vi "Build Msgs.vi"(8 "error in (no error)":errorcluster, 9 "Messages in":map{string, T3}(c390), 10 "Segments in":T1[](array[typedef]), 11 "ProtoParser in":refnum<class "ProtoParser.lvclass">) -> (0 "error out":errorcluster, 1 "Messages":map{string, T3}(c390), 2 "Segments":T1[](array[typedef]), 3 "ProtoParser out":refnum<class "ProtoParser.lvclass">)   [LabVIEW 2020, in "LV-Protoc.lvlib" / "ProtoParser.lvclass"]
uses:
  ProtoParser.lvclass
  Segment Type.ctl
  LV-Protoc.lvlib
  Raw Segment.ctl
  LV-Proto/Proto Type.ctl
  LV-Proto/LV-Proto.lvlib
  LV-Proto/Field.ctl
  LV-Proto/Message.ctl
  LV-Proto/Type.ctl
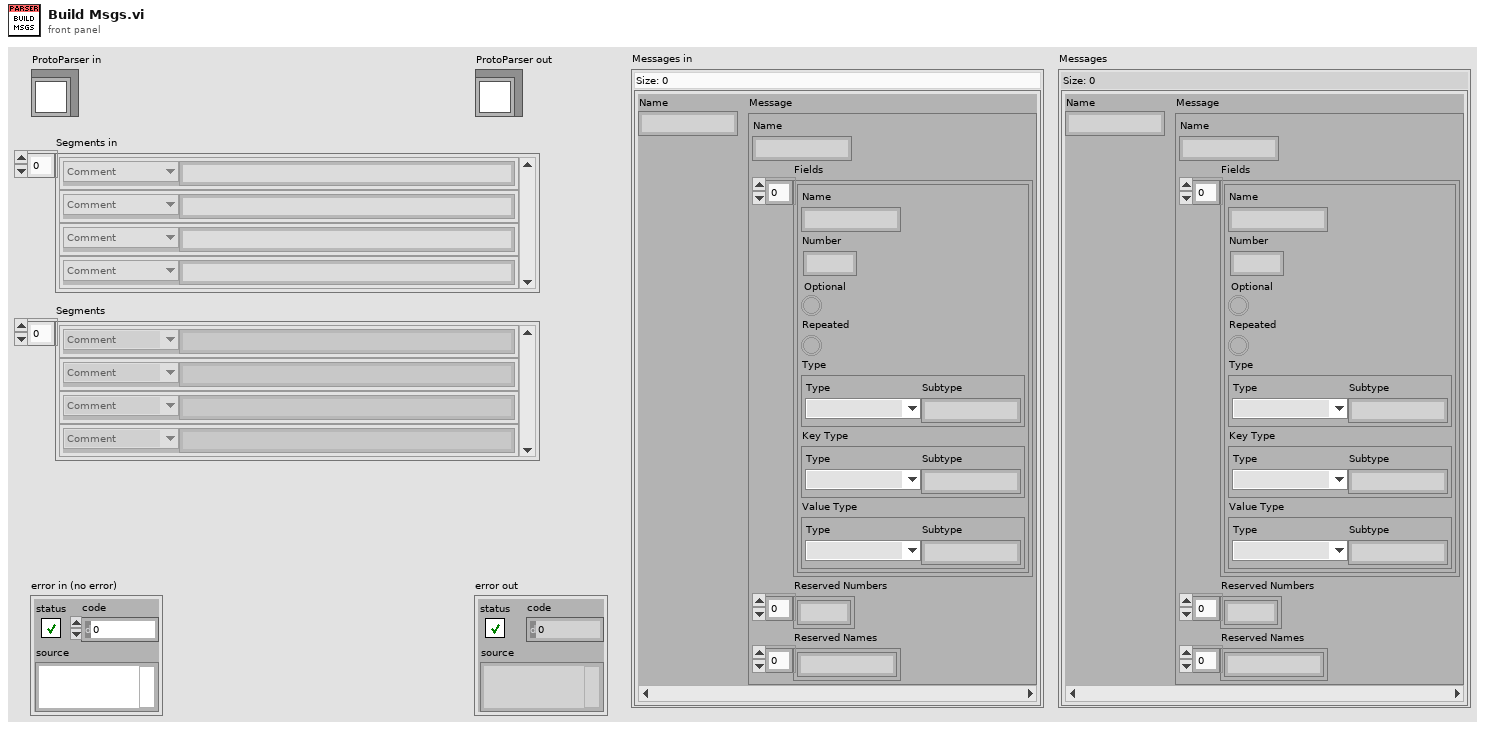
[diagram p1: front panel]
types:
  T1 = typedef "LV-Protoc.lvlib/Raw Segment.ctl" = cluster{"Type":T2, "Text":string}
  T2 = typedef "LV-Protoc.lvlib/Segment Type.ctl" = enum16{"Comment", "Message Open", "Enum Open", "Message Close", "Enum Close", "Field", "Syntax", "Import", "Enum Value", "Package", "Reserved"}
  T3 = typedef "LV-Proto.lvlib/Message.ctl" = cluster{"Name":string, "Fields":T4[], "Reserved Numbers":u32[], "Reserved Names":string[]}
  T4 = typedef "LV-Proto.lvlib/Field.ctl" = cluster{"Name":string, "Number":u32, "Optional":bool, "Repeated":bool, "Type":T5, "Key Type":T5, "Value Type":T5}
  T5 = typedef "LV-Proto.lvlib/Type.ctl" = cluster{"Type":T6, "Subtype":string}
  T6 = typedef "LV-Proto.lvlib/Proto Type.ctl" = enum16{"UNKNOWN", "double", "float", "int32", "int64", "uint32", "uint64", "sint32", "sint64", "fixed32", "fixed64", "sfixed32", "sfixed64", "bool", "string", "bytes", "enum", "map", "message"}
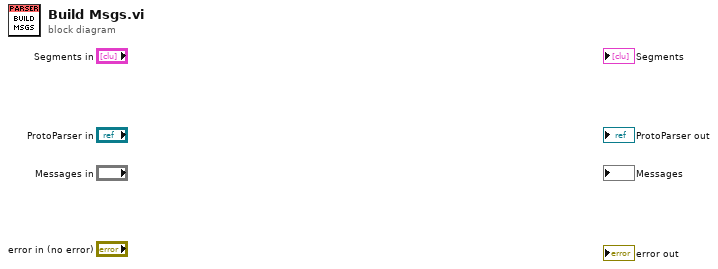
[diagram p0: block diagram]
diagram:
